vi "set PG according to private data - fast.vi"(8 "error in (no error)":errorcluster, 11 "Pulse Gen Scan in":refnum<class "Pulse Gen Scan.lvclass">) -> (0 "error out":errorcluster, 3 "Pulse Gen Scan out":refnum<class "Pulse Gen Scan.lvclass">)   [LabVIEW 2009, in "Pulse Gen Scan.lvclass"]
uses:
  Pulse Gen Scan.lvclass
  Pulse Gen Scan.lvclass/Pulse Gen Scan.ctl
  Instruments/Utility Classes/Scannable/Scannable.lvclass
panel:
  out "Outputs on/off":bool[](array[boolean])
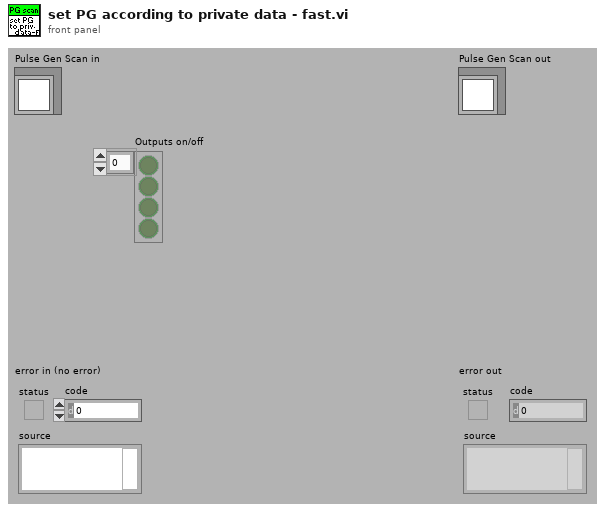
[diagram p1: front panel]
types:
  T1 = enum16{"Channel All ", "Channel 1", "Channel 2", "Channel 3", "Channels Combined"}
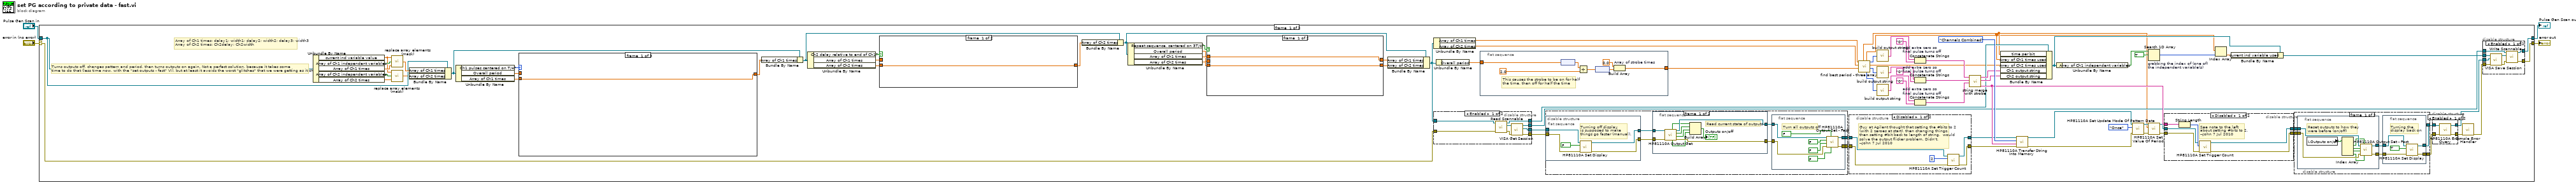
[diagram p0: block diagram]
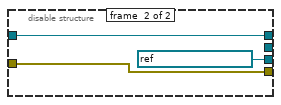
[diagram p5: hidden frame]
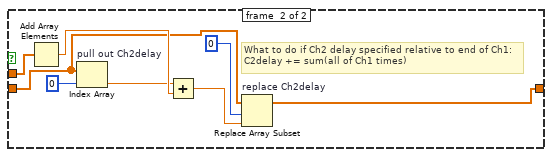
[diagram p9: hidden frame]
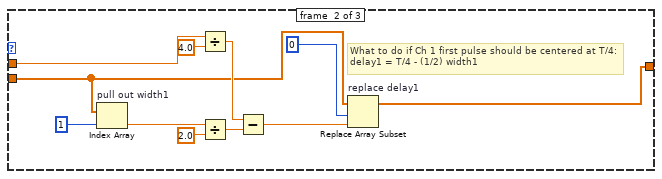
[diagram p10: hidden frame]
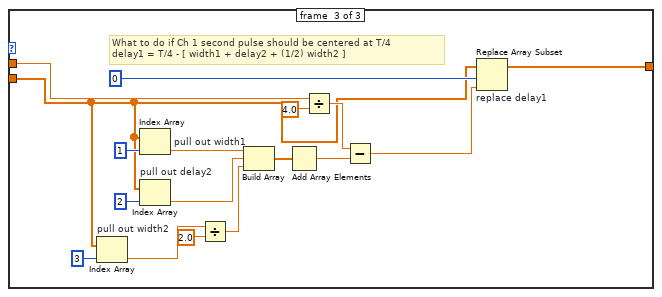
[diagram p11: hidden frame]
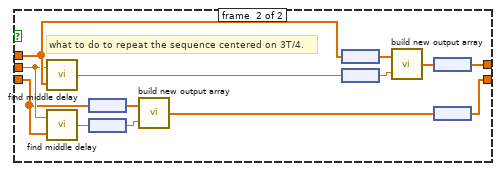
[diagram p12: hidden frame]
diagram:
  n1 = case shown="No Error" "error in (no error)" {
    selector: "error in (no error)" -> [w40 w242]
    tunnel: [w35 w242] -> w3
    tunnel: "Pulse Gen Scan in" -> [w62 w241]
    tunnel: [w33 w241] -> w1
    frame #0 {
      # "Turns outputs off, changes pattern and period, then turns outputs on again. Not a perfect solution, because it takes some \ntime to do that (less time now, with the \"set outputs - fast\" VI), but at least it avoids the worst \"glitches\" that we were getting as it changed pts."
      # "Array of Ch1 times: delay1; width1; delay2; width2; delay3; width3\nArray of Ch2 times: Ch2delay; Ch2width"
      n2 = Unbundle By Name(w62) -> ("current ind variable value"=w61:dbl[unit], "Array of Ch1 independent variables"=w67:bool[], "Array of Ch1 times"=w66:dbl[unit][], "Array of Ch2 independent variables"=w60:bool[], "Array of Ch2 times"=w59:dbl[unit][])
      n3 = call "replace array elements (mask).vi"("input array of numbers"=w66, "array of booleans (mask)"=w67, "value"=w61) -> ("output array"=w63:dbl[unit][])
      n4 = call "replace array elements (mask).vi"("input array of numbers"=w59, "array of booleans (mask)"=w60, "value"=w61) -> ("output array"=w58:dbl[unit][])
      n5 = Bundle By Name(cluster=w62, "Array of Ch1 times"=w63, "Array of Ch2 times"=w58) -> (w56:refnum<class "Pulse Gen Scan.lvclass">)
      n6 = Unbundle By Name(w56) -> ("Ch1 pulses centered on T/4?"=w81:enum32{"none", "first", "second"}, "Overall period"=w65:dbl[unit], "Array of Ch1 times"=w64:dbl[unit][])
      n7 = case shown="\"second\"" w81 {
        tunnel: w64 -> [w197 w199 w211]
        tunnel: [w197 w201 w217] -> w57
        tunnel: w65 -> [_ w202 w218]
        frame #0 {
        }
        frame #1 {
          # "What to do if Ch 1 first pulse should be centered at T/4:\ndelay1 = T/4 - (1/2) width1"
          n8 = Index Array "pull out width1"(array=w199, index=1) -> (element=w198:dbl[unit])
          n9 = Divide(x=w202, y=4.0) -> (x/y=w207:dbl[unit])
          n10 = Divide(x=w198, y=2.0) -> (x/y=w205:dbl[unit])
          n11 = Subtract(x=w207, y=w205) -> (x-y=w203:dbl[unit])
          n12 = Replace Array Subset "replace delay1"(array=w199, new element=w203, index=0) -> (w201:dbl[unit][])
        }
        frame #2 {
          # "What to do if Ch 1 second pulse should be centered at T/4\ndelay1 = T/4 - [ width1 + delay2 + (1/2) width2 ]"
          n13 = Index Array "pull out width2"(array=w211, index=3) -> (element=w210:dbl[unit])
          n14 = Index Array "pull out width1"(array=w211, index=1) -> (element=w215:dbl[unit])
          n15 = Index Array "pull out delay2"(array=w211, index=2) -> (element=w213:dbl[unit])
          n16 = Divide(x=w210, y=2.0) -> (x/y=w220:dbl[unit])
          n17 = Build Array(w215, w213, w220) -> (w222:dbl[unit][])
          n18 = Add Array Elements(numeric array=w222) -> (sum=w221:dbl[unit])
          n19 = Divide(x=w218, y=4.0) -> (x/y=w224:dbl[unit])
          n20 = Subtract(x=w224, y=w221) -> (x-y=w209:dbl[unit])
          n21 = Replace Array Subset "replace delay1"(array=w211, new element=w209, index=0) -> (w217:dbl[unit][])
        }
      }
      n22 = Bundle By Name(cluster=w56, "Array of Ch1 times"=w57) -> (w41:refnum<class "Pulse Gen Scan.lvclass">)
      n23 = Unbundle By Name(w41) -> ("Ch2 delay relative to end of Ch1?"=w51:bool, "Array of Ch1 times"=w55:dbl[unit][], "Array of Ch2 times"=w50:dbl[unit][])
      n24 = case shown="True" w51 {
        tunnel: [w188 w191] -> w54
        tunnel: w50 -> [w188 w189]
        tunnel: w55 -> [_ w195]
        frame #0 {
        }
        frame #1 {
          # "What to do if Ch2 delay specified relative to end of Ch1:\nC2delay += sum(all of Ch1 times)"
          n25 = Add Array Elements(numeric array=w195) -> (sum=w196:dbl[unit])
          n26 = Index Array "pull out Ch2delay"(array=w189, index=0) -> (element=w190:dbl[unit])
          n27 = Add(x=w190, y=w196) -> (x+y=w192:dbl[unit])
          n28 = Replace Array Subset "replace Ch2delay"(array=w189, new element=w192, index=0) -> (w191:dbl[unit][])
        }
      }
      n29 = Bundle By Name(cluster=w41, "Array of Ch2 times"=w54) -> (w47:refnum<class "Pulse Gen Scan.lvclass">)
      n30 = Unbundle By Name(w47) -> ("Repeat sequence, centered on 3T/4?"=w48:bool, "Overall period"=w49:dbl[unit], "Array of Ch1 times"=w52:dbl[unit][], "Array of Ch2 times"=w53:dbl[unit][])
      n31 = case shown="True" w48 {
        tunnel: w52 -> [w227 w234]
        tunnel: [w227 w237] -> w46
        tunnel: w53 -> [w226 w229]
        tunnel: [w226 w235] -> w45
        tunnel: w49 -> [_ w232]
        frame #0 {
        }
        frame #1 {
          # "what to do to repeat the sequence centered on 3T/4."
          n32 = call "find middle delay.vi"("array of times"=w234, "Expected overall period"=w232) -> ("middle delay"=w233:dbl[unit])
          n33 = call "find middle delay.vi"("array of times"=w229, "Expected overall period"=w232) -> ("middle delay"=w231:dbl[unit])
          n34 = node(w229) -> (w228:dbl[])
          n35 = node(w231) -> (w230:dbl)
          n36 = call "build new output array.vi"("number to insert"=w230, "input array"=w228) -> ("output array"=w236:dbl[])
          n37 = node(w234) -> (w240:dbl[])
          n38 = node(w233) -> (w239:dbl)
          n39 = call "build new output array.vi"("number to insert"=w239, "input array"=w240) -> ("output array"=w238:dbl[])
          n40 = node(w238) -> (w237:dbl[unit][])
          n41 = node(w236) -> (w235:dbl[unit][])
        }
      }
      n42 = Bundle By Name(cluster=w47, "Array of Ch1 times"=w46, "Array of Ch2 times"=w45) -> (w9:refnum<class "Pulse Gen Scan.lvclass">)
      n43 = Unbundle By Name(w9) -> ("Array of Ch1 times"=w18:dbl[unit][], "Array of Ch2 times"=w17:dbl[unit][])
      n44 = disable-structure shown="Enabled" {
        disable-tunnel: w40 -> [w161 w165]
        disable-tunnel: [w160 w166] -> w39
        disable-tunnel: w9 -> [w159 w166]
        disable-tunnel: [w158 _] -> w37
        disable-tunnel: [w157 refnum<visa-resource-name> "GPIB0::10::INSTR" ("VISA Resource Name")] -> w32
        disable-tunnel: [w156 w165] -> w31
        frame #0 {
          n45 = call-dynamic "Read Scannable.vi"("error in (no error)"=w161, "Scanner.lvclass in"=w159) -> ("error out"=w162:errorcluster, "Scannable.lvclass"=w163:refnum<class "Scannable.lvclass">, "Scanner.lvclass out"=w160:refnum<class "Pulse Gen Scan.lvclass">)  [unwired: 7 out]
          n46 = call-dynamic "VISA Get Session.vi"("error in (no error)"=w162, "Instrument.lvclass in"=w163) -> ("error out"=w156:errorcluster, "VISA Resource Name"=w157:refnum<visa-resource-name>, "Instrument.lvclass out"=w158:refnum<class "Scannable.lvclass">)  [unwired: 7 out]
        }
        frame #1 {
        }
      }
      n47 = Unbundle By Name(w9) -> ("Overall period"=w8:dbl[unit])
      n48 = flat-sequence {
        tunnel: [w142] -> w16
        tunnel: w8 -> [w141]
        frame #0 {
          # "This causes the strobe to be on for half the time, then off for half the time"
          n49 = node(w141) -> (w145:dbl)
          n50 = Divide(x=w145, y=2.0) -> (x/y=w143:dbl)
          n51 = node(w143) -> (w140:dbl[unit])
          n52 = Build Array "Array of strobe times"(dbl[unit] 0.0 ("element"), w140) -> (w142:dbl[unit][])
        }
      }
      n53 = disable-structure shown="Enabled" {
        disable-tunnel: w32 -> [w112 w138]
        disable-tunnel: w31 -> [w110 w137]
        disable-tunnel: [w108 w138] -> w30
        disable-tunnel: [w107 w137] -> w29
        frame #0 {
          n54 = flat-sequence {
            tunnel: w112 -> [w118]
            tunnel: [w117] -> w111
            tunnel: w110 -> [w116]
            tunnel: [w115] -> w109
            frame #0 {
              # "Turning off display\nis supposed to make \nthings go faster (manual)."
              n55 = call "HP81110A Set Display.vi"("error in (no error)"=w116, "Display (F:Off)"=FALSE, "VISA session"=w118) -> ("error out"=w115:errorcluster, "dup VISA session"=w117:refnum<visa-resource-name>)  [unwired: 7 out]
            }
          }
          n56 = flat-sequence {
            tunnel: [w136] -> w114
            tunnel: [w135] -> w113
            tunnel: w109 -> [w134]
            tunnel: w111 -> [w133]
            frame #0 {
              # "Read current state of outputs"
              n57 = call "HP81110A Output Get.vi"("error in (no error)"=w134, "VISA session"=w133) -> ("error out"=w135:errorcluster, "output2OUT"=w130:bool, "notoutput1OUT"=w131:bool, "dup VISA session"=w136:refnum<visa-resource-name>, "notoutput2OUT"=w129:bool, "output1OUT"=w132:bool)  [unwired: 4 out]
              n58 = Build Array(w132, w131, w130, w129) -> (→"Outputs on/off":bool[])
            }
          }
          n59 = flat-sequence {
            tunnel: w114 -> [w127]
            tunnel: w113 -> [w126]
            tunnel: [w125] -> w108
            tunnel: [w124] -> w107
            frame #0 {
              # "Turn all outputs off"
              n60 = call "HP81110A Output Set - Fast.vi"("notoutput2"=FALSE, "output1"=FALSE, "error in (no error)"=w126, "output2"=FALSE, "notoutput1"=FALSE, "VISA session"=w127) -> ("error out"=w124:errorcluster, "dup VISA session"=w125:refnum<visa-resource-name>)  [unwired: 4 out]
            }
          }
        }
        frame #1 {
        }
      }
      n61 = disable-structure shown="Disabled" {
        disable-tunnel: w30 -> [w178 w181]
        disable-tunnel: w29 -> [w177 w180]
        disable-tunnel: [w176 w180] -> w23
        disable-tunnel: [w175 w181] -> w24
        frame #0 {
          # "Guy at Agilent thought that setting the #bits to 2 \n(with 2 zeroes at start), then changing things, \nthen setting #bit back to length of string,  would \nsolve the output flicker problem. Didn't.\n--John 7 Jul 2010"
          n62 = call "HP81110A Set Trigger Count.vi"("error in (no error)"=w177, "Trigger Count"=2, "VISA session"=w178) -> ("error out"=w176:errorcluster, "dup VISA session"=w175:refnum<visa-resource-name>)  [unwired: 7 out]
        }
        frame #1 {
        }
      }
      n63 = call "find best period - three array.vi"("Array of strobe desired times"=w16, "Array of Ch2 desired times"=w17, "Array of Ch1 desired times"=w18) -> ("Array of Ch2 \"period-units\""=w11:i32[], "Array of Ch2 actual times"=w12:dbl[unit][], "Array of Ch1 \"period-units\""=w13:i32[], "Array of strobe \"period-units\""=w10:i32[], "Array of Ch1 actual times"=w14:dbl[unit][], "best period"=w15:dbl[unit])  [unwired: 2 in, 1 out]
      n64 = call "build output string.vi"("Array of \"period-units\""=w13) -> ("output string"=w77:string)
      n65 = call "build output string.vi"("Array of \"period-units\""=w11) -> ("output string"=w76:string)
      n66 = call "build output string.vi"("Array of \"period-units\""=w10) -> ("output string"=w6:string)
      n67 = Concatenate Strings "add extra zero so \nfinal pulse turns off"(w77, "0" ("string")) -> (w73:string)
      n68 = Concatenate Strings "add extra zero so \nfinal pulse turns off"(w76, "0" ("string")) -> (w72:string)
      n69 = Concatenate Strings "add extra zero so \nfinal pulse turns off"(w6, "0" ("string")) -> (w5:string)
      n70 = call "string merge with strobe.vi"("Strobe String"=w5, "Ch2 String"=w72, "Ch1 String"=w73) -> ("Merged Output String"=w68:string, "Ch2 Output String"=w42:string, "Ch1 Output String"=w43:string)  [unwired: 5 in, 1 out]
      n71 = Bundle By Name(cluster=w39, "time per bit"=w15, "Array of Ch1 times used"=w14, "Array of Ch2 times used"=w12, "Ch1 output string"=w43, "Ch2 output string"=w42) -> (w44:refnum<class "Pulse Gen Scan.lvclass">)
      n72 = call "HP81110A Transfer String Into Memory.vi"("error in (no error)"=w23, "String"=w68, "Channel (1:Channel 1)"=T1."Channels Combined", "VISA session"=w24) -> ("error out"=w69:errorcluster, "dup VISA session"=w70:refnum<visa-resource-name>)  [unwired: 6 out]
      n73 = Unbundle By Name(w44) -> ("Array of Ch1 independent variables"=w83:bool[])
      n74 = call "HP81110A Set Update Mode Of Pattern Data.vi"("error in (no error)"=w69, "Pattern Update Mode (1:Continuous)"=enum16{"Off", "Continuous", "Once"}."Once", "VISA session"=w70) -> ("error out"=w26:errorcluster, "dup VISA session"=w28:refnum<visa-resource-name>)  [unwired: 7 out]
      n75 = Search 1D Array "grabbing the index of (one of) \nthe independent variable(s)"(1D array=w83, element=TRUE) -> (index of element=w82:i32)  [unwired: 1 out]
      n76 = call "HP81110A Set Value Of Period.vi"("error in (no error)"=w26, "Period Value"=w15, "VISA session"=w28) -> ("error out"=w25:errorcluster, "dup VISA session"=w27:refnum<visa-resource-name>)  [unwired: 7 out]
      n77 = disable-structure shown="Disabled" {
        disable-tunnel: [w171 w174] -> w20
        disable-tunnel: [w170 w173] -> w19
        disable-tunnel: w27 -> [w169 w174]
        disable-tunnel: w25 -> [w168 w173]
        disable-tunnel: w68 -> [w167 _]
        frame #0 {
          # "See note to the left \nabout setting #bits to 2.\n--John 7 Jul 2010"
          n78 = String Length(string=w167) -> (length=w172:i32)
          n79 = call "HP81110A Set Trigger Count.vi"("error in (no error)"=w168, "Trigger Count"=w172, "VISA session"=w169) -> ("error out"=w170:errorcluster, "dup VISA session"=w171:refnum<visa-resource-name>)  [unwired: 7 out]
        }
        frame #1 {
        }
      }
      n80 = Index Array(array=w14, index=w82) -> (element=w80:dbl[unit])
      n81 = Bundle By Name(cluster=w44, "current ind variable used"=w80) -> (w34:refnum<class "Pulse Gen Scan.lvclass">)
      n82 = disable-structure shown="Enabled" {
        disable-tunnel: [w90 w106] -> w22
        disable-tunnel: [w88 w105] -> w21
        disable-tunnel: w20 -> [w86 w106]
        disable-tunnel: w19 -> [w85 w105]
        frame #0 {
          n83 = flat-sequence {
            tunnel: [w104] -> w89
            tunnel: [w103] -> w87
            tunnel: w86 -> [w102]
            tunnel: w85 -> [w101]
            frame #0 {
              # "Reset outputs to how they \nwere before (on/off)"
              n84 = local read "Outputs on/off"() -> (w100:bool[])
              n85 = Index Array(array=w100) -> (element #1=w99:bool, element #2=w98:bool, element #3=w97:bool, element #4=w96:bool)  [unwired: 4 in]
              n86 = call "HP81110A Output Set - Fast.vi"("notoutput2"=w96, "output1"=w99, "error in (no error)"=w101, "output2"=w97, "notoutput1"=w98, "VISA session"=w102) -> ("error out"=w103:errorcluster, "dup VISA session"=w104:refnum<visa-resource-name>)  [unwired: 4 out]
            }
          }
          n87 = flat-sequence {
            tunnel: [w94] -> w90
            tunnel: w89 -> [w93]
            tunnel: [w92] -> w88
            tunnel: w87 -> [w91]
            frame #0 {
              # "Turning the \ndisplay back on"
              n88 = call "HP81110A Set Display.vi"("error in (no error)"=w91, "Display (F:Off)"=TRUE, "VISA session"=w93) -> ("error out"=w92:errorcluster, "dup VISA session"=w94:refnum<visa-resource-name>)  [unwired: 7 out]
            }
          }
        }
        frame #1 {
        }
      }
      n89 = disable-structure shown="Enabled" {
        disable-tunnel: [w185 w187] -> w74
        disable-tunnel: w22 -> [w184 w186]
        disable-tunnel: w21 -> [w183 w187]
        disable-tunnel: [w182 w186] -> w38
        frame #0 {
          n90 = call "HP81110A Error Query.vi"("VISA session"=w184, "error in (no error)"=w183) -> ("dup VISA session"=w182:refnum<visa-resource-name>, "error out"=w185:errorcluster)  [unwired: 12 out]
        }
        frame #1 {
        }
      }
      n91 = call <vilib>:"Simple Error Handler.vi"("error in (no error)"=w74) -> ("error out"=w36:errorcluster)  [unwired: 1 in, 7 out]
      n92 = disable-structure shown="Enabled" {
        disable-tunnel: w38 -> [w153 _]
        disable-tunnel: w37 -> [w152 _]
        disable-tunnel: w36 -> [w150 w154]
        disable-tunnel: [w149 w154] -> w35
        disable-tunnel: w34 -> [w148 w155]
        disable-tunnel: [w147 w155] -> w33
        frame #0 {
          n93 = call-dynamic "VISA Save Session.vi"("error in (no error)"=w150, "VISA Resource Name"=w153, "Instrument.lvclass in"=w152) -> ("error out"=w151:errorcluster, "Instrument.lvclass out"=w146:refnum<class "Scannable.lvclass">)  [unwired: 7 out]
          n94 = call-dynamic "Write Scannable.vi"("error in (no error)"=w151, "Scannable.lvclass"=w146, "Scanner.lvclass in"=w148) -> ("error out"=w149:errorcluster, "Scanner.lvclass out"=w147:refnum<class "Pulse Gen Scan.lvclass">)  [unwired: 7 out]
        }
        frame #1 {
        }
      }
    }
    frame #1 {
    }
  }
  "error out" <- w3
  "Pulse Gen Scan out" <- w1
